vi "lab1_packet_parser.vi"(10 "preamble bytes":u8[](array[numeric]), 11 "bitstream":i16[](array[numeric])) -> (0 "Found?":bool, 1 "packet counter":u32, 2 "payload length(bytes)":u32, 3 "payload bytes":u8[](array[numeric]))   [LabVIEW 2014]
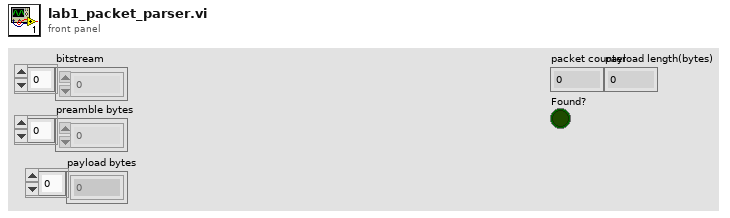
[diagram p1: front panel]
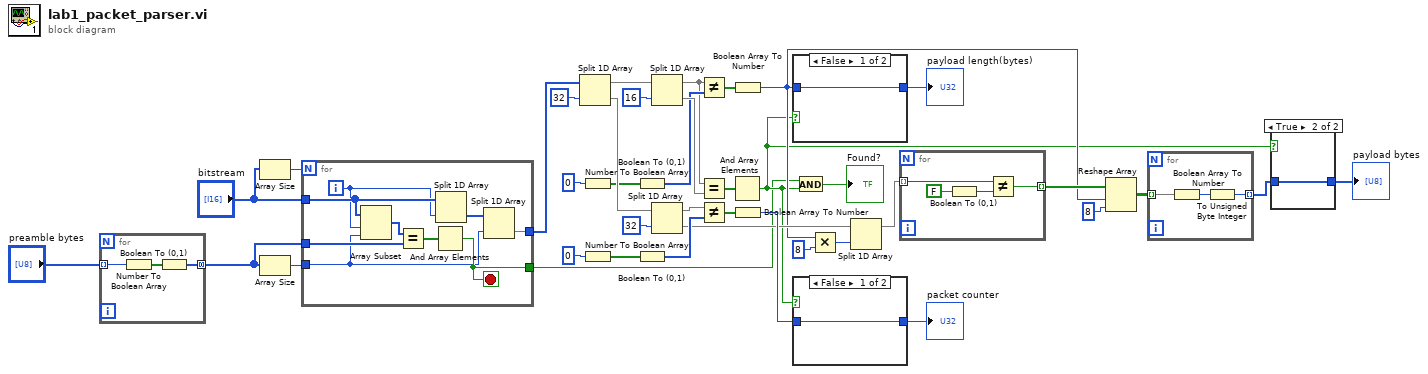
[diagram p0: block diagram]
diagram:
  n1 = for {
    tunnel: "preamble bytes" -> [w42] mode=indexing
    tunnel: [w40] -> w17 mode=concatenating
    n2 = Number To Boolean Array(number=w42) -> (Boolean array=w41:bool[])
    n3 = Boolean To (0,1)(Boolean=w41) -> (0, 1=w40:i16[])
  }
  n4 = Array Size(array="bitstream") -> (size(s)=w14:i32)
  n5 = Array Size(array=w17) -> (size(s)=w16:i32)
  n6 = for {
    N: w14 -> [_]
    tunnel: "bitstream" -> [w47]
    tunnel: w17 -> [w51]
    tunnel: w16 -> [w44]
    tunnel: [w43] -> w15
    tunnel: [w48] -> w1
    i -> [w45]
    stop <- w48 stop-if-true
    n7 = Array Subset(array=w47, index=w45, length=w44) -> (w49:i16[])
    n8 = Equal?(x=w49, y=w51) -> (x = y?=w50:bool[])
    n9 = And Array Elements(Boolean array=w50) -> (logical AND=w48:bool)
    n10 = Split 1D Array(array=w47, index=w45) -> (second subarray=w46:i16[])  [unwired: 1 out]
    n11 = Split 1D Array(array=w46, index=w44) -> (second subarray=w43:i16[])  [unwired: 1 out]
  }
  n12 = Split 1D Array(array=w15, index=u8 32) -> (first subarray=w37:i16[], second subarray=w34:i16[])
  n13 = Number To Boolean Array(number=u16 0) -> (Boolean array=w31:bool[])
  n14 = Number To Boolean Array(number=u32 0) -> (Boolean array=w26:bool[])
  n15 = Boolean To (0,1)(Boolean=w31) -> (0, 1=w30:i16[])
  n16 = Boolean To (0,1)(Boolean=w26) -> (0, 1=w25:i16[])
  n17 = Split 1D Array(array=w37, index=u8 16) -> (first subarray=w20:i16[], second subarray=w36:i16[])
  n18 = Split 1D Array(array=w34, index=u8 32) -> (first subarray=w24:i16[], second subarray=w11:i16[])
  n19 = Not Equal?(x=w20, y=w30) -> (x != y?=w29:bool[])
  n20 = Equal?(x=w20, y=w36) -> (x = y?=w35:bool[])
  n21 = Not Equal?(x=w24, y=w25) -> (x != y?=w23:bool[])
  n22 = And Array Elements(Boolean array=w35) -> (logical AND=w2:bool)
  n23 = Boolean Array To Number(Boolean array=w29) -> (number=w5:u32)
  n24 = Boolean Array To Number(Boolean array=w23) -> (number=w22:u32)
  n25 = case shown="False" w2 {
    tunnel: w5 -> [w52 w53]
    tunnel: [w52 w53] -> w19
    frame False {
    }
    frame True {
    }
  }
  "payload length(bytes)" <- w19
  n26 = case shown="False" w2 {
    tunnel: w22 -> [w54 w55]
    tunnel: [w54 w55] -> w21
    frame False {
    }
    frame True {
    }
  }
  "packet counter" <- w21
  n27 = And(x=w1, y=w2) -> (x .and. y?=→"Found?":bool)
  n28 = Multiply(x=w5, y=8) -> (x*y=w18:u32)
  n29 = Split 1D Array(array=w11, index=w18) -> (first subarray=w10:i16[])  [unwired: 1 out]
  n30 = for {
    tunnel: w10 -> [w59] mode=indexing
    tunnel: [w58] -> w9 mode=indexing
    n31 = Boolean To (0,1)(Boolean=FALSE) -> (0, 1=w56:i16)
    n32 = Not Equal?(x=w59, y=w56) -> (x != y?=w58:bool)
  }
  n33 = Reshape Array(w9, w5, 8) -> (w8:bool[][])
  n34 = for {
    tunnel: w8 -> [w61] mode=indexing
    tunnel: [w60] -> w7 mode=indexing
    n35 = Boolean Array To Number(Boolean array=w61) -> (number=w62:u32)
    n36 = To Unsigned Byte Integer(number=w62) -> (unsigned 8bit integer=w60:u8)
  }
  n37 = case shown="True" w2 {
    tunnel: w7 -> [w63 w64]
    tunnel: [w63 w64] -> w6
    frame False {
    }
    frame True {
    }
  }
  "payload bytes" <- w6
